vi "Write Enum U8.vi"(8 "error in (no error)":errorcluster, 10 "Enum U8":enum8{"One", "Two", "Three"}(ring), 11 "Numeric Types in":refnum<class "Numeric Types.lvclass">) -> (0 "error out":errorcluster, 3 "Numeric Types out":refnum<class "Numeric Types.lvclass">)   [LabVIEW 2017, in "Generic Object Serializer Tests.lvlib" / "Numeric Types.lvclass"]
uses:
  Numeric Types.lvclass
  Numeric Types.lvclass/Numeric Types.ctl
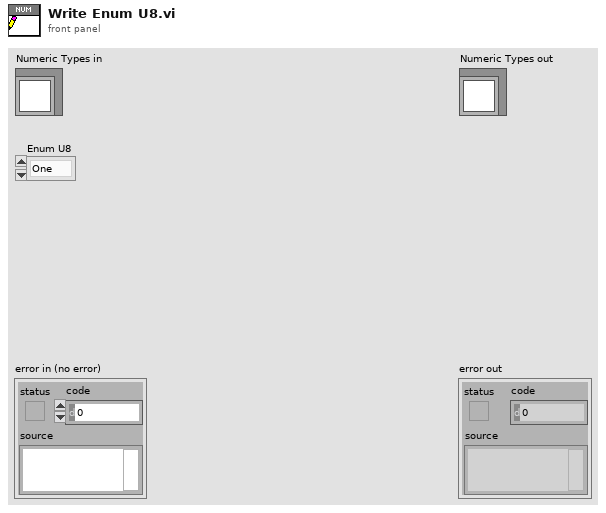
[diagram p1: front panel]
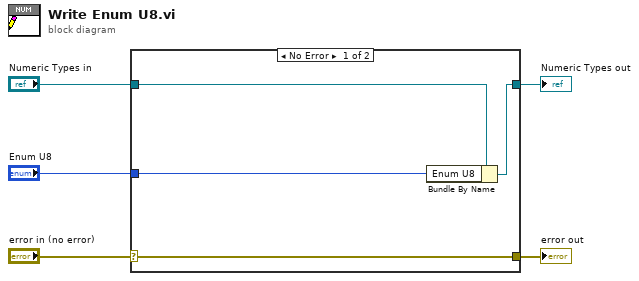
[diagram p0: block diagram]
diagram:
  n1 = case shown="No Error" "error in (no error)" {
    selector: "error in (no error)" -> [w9 w10]
    tunnel: [w9 w10] -> w4
    tunnel: [w7 w11] -> w2
    tunnel: "Numeric Types in" -> [w8 w11]
    tunnel: "Enum U8" -> [w6 _]
    frame No Error {
      n2 = Bundle By Name(cluster=w8, "Enum U8"=w6) -> (w7:refnum<class "Numeric Types.lvclass">)
    }
    frame Error {
    }
  }
  "error out" <- w4
  "Numeric Types out" <- w2
